vi "Periodic Tasks.vi"(8 "error in":errorcluster) -> ()   [LabVIEW 2016]
doc: "This VI runs in parallel to other tasks. It can contain as many user-defined periodic loops as you need. These can carry out PID or other sorts of timed response."
uses:
  <vilib>/Rock Robotics/WPI/DriverStation/WPI_DriverStationRobotMode2.ctl
  <vilib>/Rock Robotics/WPI/Utilities/WPI_GetSetVariantRefNum.vi
  Robot Global Data.vi
  AutoLeftDrive.vi
  AutoRightDrive.vi
  Target x Location.vi
  AutoModEnable.vi
  AutoProceed.vi
  AutoMod.vi
  <vilib>/Rock Robotics/Network Tables/NT Write Number.vi
  <vilib>/Rock Robotics/WPI/Ultrasonic/WPI_SonarSRF04DigitalRefNum Registry Get.vi
  <vilib>/Rock Robotics/WPI/Ultrasonic/WPI_SonarSRF04DigitalGetRange.vi
panel:
  out "Auto Mod Enable":bool
  out "Target x Location contr":dbl
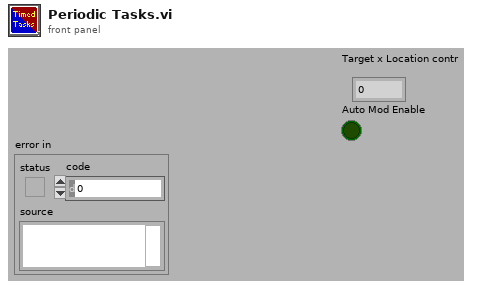
[diagram p1: front panel]
types:
  T1 = typedef "WPI_JoystickDevRef.ctl" = cluster{"Device":T2}
  T2 = typedef "WPI_JoystickDeviceEnum.ctl" = enum16{"USB 0", "USB 1", "USB 2", "USB 3", "USB 4", "USB 5"}
  T3 = typedef "WPI_RobotDriveDevRef.ctl" = cluster{"DevStatus":errorcluster, "Motors[]":T4[], "Square Inputs":bool, "Max Output":dbl}
  T4 = typedef "WPI_MotorControlDeviceRef.ctl" = cluster{"DeviceStatus":errorcluster, "Type":T5, "PWM":cluster{"PWM Channel":T6, "DeadBand":T7}, "CAN":cluster{"Device Number":u8, "SetOutput VI Ref":variant, "GetOutput VI Ref":variant, "Enable VI Ref":variant, "Disable VI Ref":variant, "Data":variant}, "Invert":bool}
  T5 = typedef "WPI_MotorControlType.ctl" = enum16{"PWM", "CAN"}
  T6 = typedef "FPGA_DIOPWMChannel.ctl" = enum8{"PWM 0", "PWM 1", "PWM 2", "PWM 3", "PWM 4", "PWM 5", "PWM 6", "PWM 7", "PWM 8", "PWM 9", "PWM MXP 0", "PWM MXP 1", "PWM MXP 2", "PWM MXP 3", "PWM MXP 4", "PWM MXP 5", "PWM MXP 6", "PWM MXP 7", "PWM MXP 8", "PWM MXP 9", "Invalid"}
  T7 = typedef "WPI_PWMDeadband.ctl" = cluster{"Name":string, "maxPositivePwm":i32, "minPositivePwm":i32, "centerPwm":i32, "maxNegativePwm":i32, "minNegativePwm":i32, "angularRange":u16}
  T8 = typedef "WPI_DriverStationRobotMode2.ctl" = enum16{"Autonomous Disabled", "Autonomous Enabled", "Teleop Disabled", "Teleop Enabled", "Disconnected", "Finish", "Test Disabled", "Test Enabled", "Emergency Stopped"}
  T9 = cluster{"JoystickDevRef":T1, "RobotDriveDevRef":T3}
  T10 = typedef "WPI_GyroDevRef.ctl" = cluster{"DevStatus":errorcluster, "Analog Channel":T11, "Offset":dbl, "Gain (VoltsPerDegree/Second)":dbl, "Gyro Type":enum16{"Analog", "XRS450"}, "Handle":i32, "SPI Bus":T12, "Device Found":bool, "Sample Rate":dbl, "Calibrate On Open":bool}
  T11 = typedef "FPGA_AIChannel.ctl" = enum8{"AI 0", "AI 1", "AI 2", "AI 3", "AI MXP 0", "AI MXP 1", "AI MXP 2", "AI MXP 3", "Invalid"}
  T12 = typedef "spi_bus.ctl" = enum16{"SPI On-Board, CS0", "SPI On-Board, CS1", "SPI On-Board, CS2", "SPI On-Board, CS3", "SPI MXP", "Invalid"}
  T13 = typedef "WPI_UltrasonicDeviceRef.ctl" = cluster{"DevStatus":errorcluster, "Ping Channel":T14, "Echo Channel":T14, "CntIndex":T15}
  T14 = typedef "FPGA_DIOChannel.ctl" = enum8{"DIO 0", "DIO 1", "DIO 2", "DIO 3", "DIO 4", "DIO 5", "DIO 6", "DIO 7", "DIO 8", "DIO 9", "DIO MXP 0", "DIO MXP 1", "DIO MXP 2", "DIO MXP 3", "DIO MXP 4", "DIO MXP 5", "DIO MXP 6", "DIO MXP 7", "DIO MXP 8", "DIO MXP 9", "DIO MXP 10", "DIO MXP 11", "DIO MXP 12", "DIO MXP 13", "DIO MXP 14", "DIO MXP 15", "SPI Port CS1", "SPI Port CS2", "SPI Port CS3", "SPI Port MISO", "SPI Port MOSI", "Invalid"}
  T15 = typedef "FPGA_CounterCtrSystemIndex.ctl" = enum8{"Ctr 0", "Ctr 1", "Ctr 2", "Ctr 3", "Ctr 4", "Ctr 5", "Ctr 6", "Ctr 7", "Invalid"}
  T16 = typedef "WPI_EncoderDevRef.ctl" = cluster{"DevStatus":errorcluster, "EncoderIndex":T17, "CounterIndex":T15, "DistancePerCount":dbl, "Decoding Type":T18}
  T17 = typedef "FPGA_EncoderIdx.ctl" = enum8{"Enc 0", "Enc 1", "Enc 2", "Enc 3", "Enc 4", "Enc 5", "Enc 6", "Enc 7", "Invalid"}
  T18 = typedef "WPI_EncoderType.ctl" = enum16{"1x", "2x", "4x"}
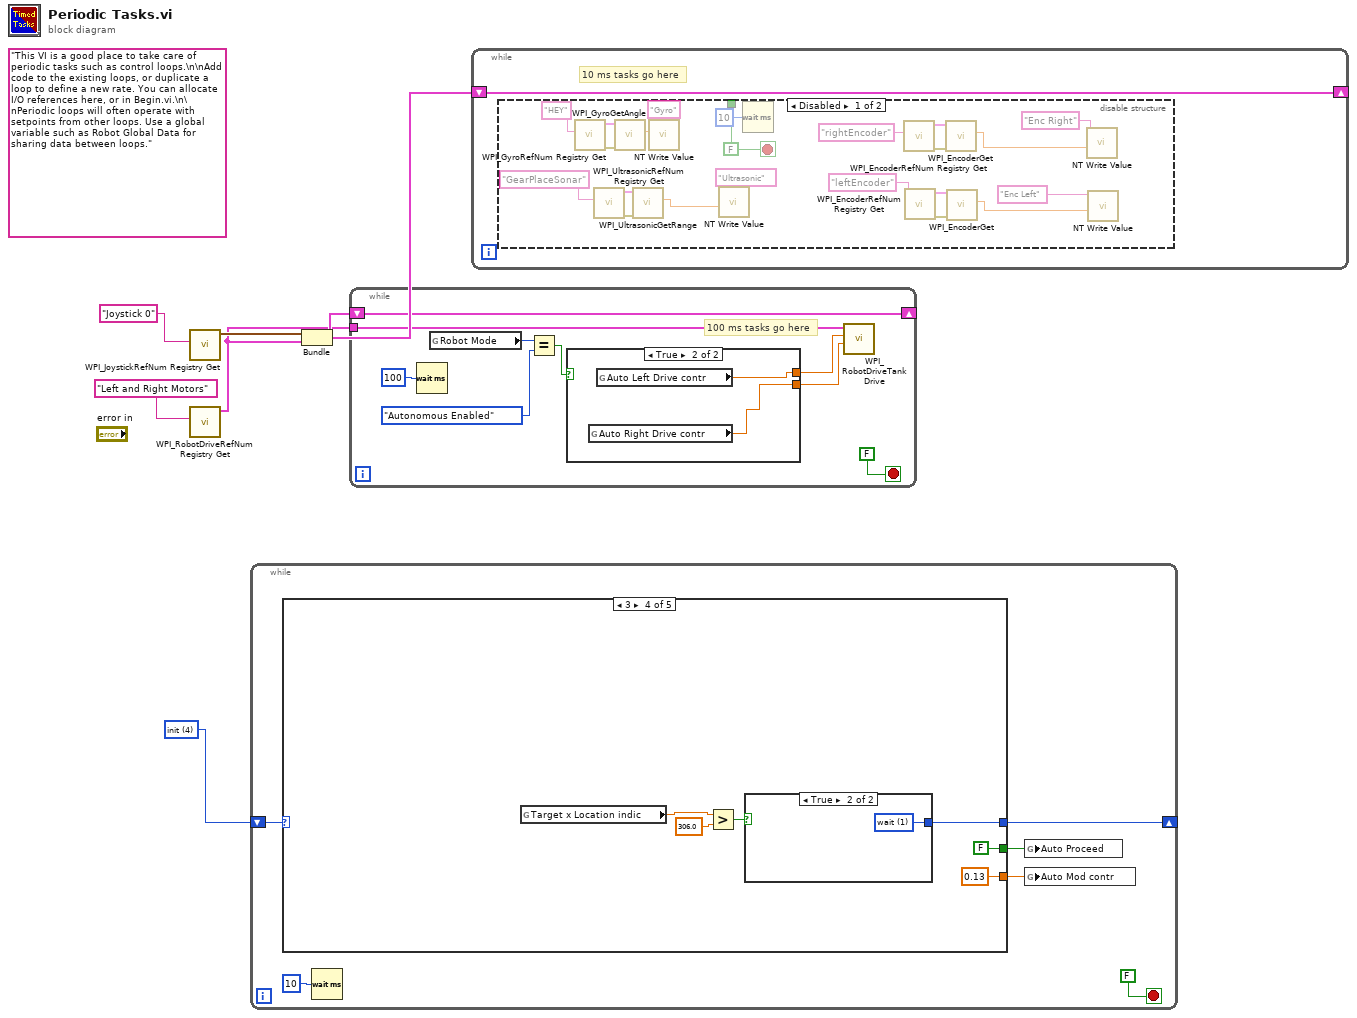
[diagram p0: block diagram]
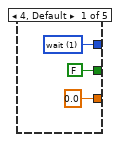
[diagram p2: hidden frame]
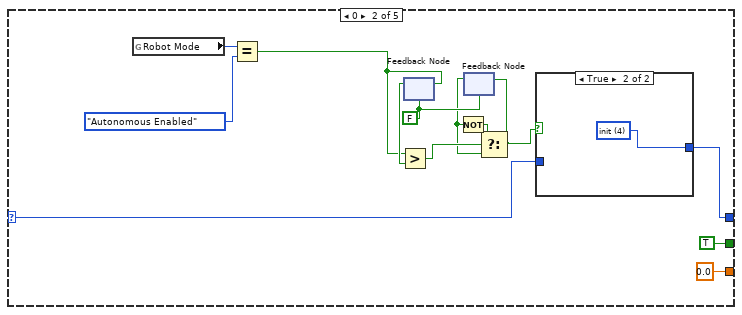
[diagram p3: hidden frame]
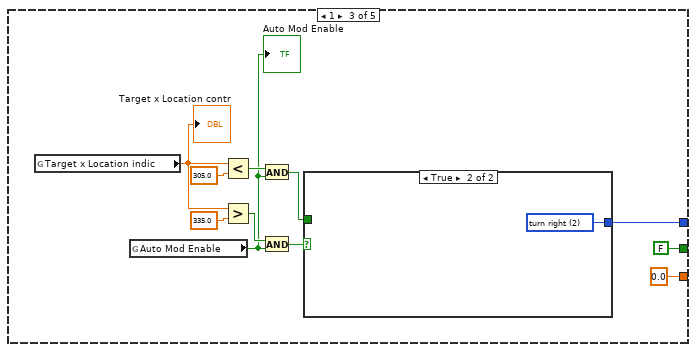
[diagram p5: hidden frame]
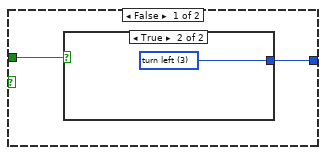
[diagram p6: hidden frame]
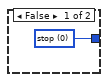
[diagram p7: hidden frame]
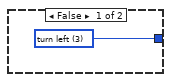
[diagram p8: hidden frame]
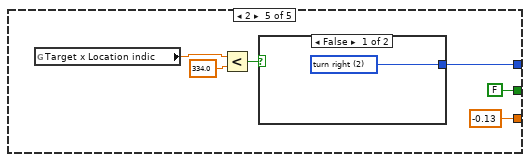
[diagram p9: hidden frame]
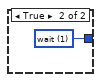
[diagram p10: hidden frame]
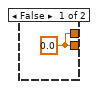
[diagram p11: hidden frame]
diagram:
  w2 = u16 4 items=["stop", "wait", "turn right", "turn left", "init"]
  (unwired) "This VI is a good place to take care of periodic tasks such as control loops.\n\nAdd code to the existing loops, or duplicate a loop to define a new rate. You can allocate I/O references here, or in Begin.vi.\n\nPeriodic loops will often operate with setpoints from other loops. Use a global variable such as Robot Global Data for sharing data between loops."
  n1 = call <vilib>:"WPI_JoystickRefNum Registry Get.vi"("refnum name"="Joystick 0") -> ("JoystickDevRef"=w4:T1)  [unwired: 1 in, 9 out]
  n2 = call <vilib>:"WPI_RobotDriveRefNum Registry Get.vi"("refnum name"="Left and Right Motors") -> ("RobotDriveDevRef"=w1:T3)  [unwired: 1 in, 9 out]
  n3 = while {
    shift-right: [w8] -> _
    shift-left: w2 -> [w7]
    stop <- FALSE stop-if-true
    n4 = case shown="3" w7 {
      selector: w7 -> [_ w16 _ _ _]
      tunnel: [0.0 0.0 0.0 0.13 -0.13] -> w10
      tunnel: [FALSE TRUE FALSE FALSE FALSE] -> w9
      tunnel: [w13 w17 w33 w49 w57] -> w8
      frame 4, Default {
        w13 = u16 1 items=["stop", "wait", "turn right", "turn left", "init"]
      }
      frame 0 {
        w22 = FALSE ("Boolean")
        n5 = global read "Robot Global Data.vi" "Robot Mode"() -> (w25:T8)
        n6 = Equal?(x=w25, y=WPI_DriverStationRobotMode2."Autonomous Enabled" ("Robot Mode")) -> (x = y?=w19:bool)
        n7 = feedback #1(w22) -> (w24:bool)
        n8 = Greater?(x=w19, y=w24) -> (0:w23:bool)
        n9 = feedback-in #1(w19) -> ()
        n10 = feedback #2(w22) -> (w21:bool)
        n11 = Not(x=w21) -> (.not. x?=w20:bool)
        n12 = Select(t=w20, s=w23, f=w21) -> (s? t:f=w18:bool)
        n13 = feedback-in #2(w18) -> ()
        n14 = case shown="True" w18 {
          tunnel: [w29 w30] -> w17
          tunnel: w16 -> [w29 _]
          frame False {
          }
          frame True {
            w30 = u16 4 items=["stop", "wait", "turn right", "turn left", "init"]
          }
        }
      }
      frame 1 {
        n15 = global read "Target x Location.vi" "Target x Location indic"() -> (w40:dbl)
        "Target x Location contr" <- w40
        n16 = global read "AutoModEnable.vi" "Auto Mod Enable"() -> (w36:bool)
        "Auto Mod Enable" <- w36
        n17 = Less?(x=w40, y=305.0) -> (x < y?=w37:bool)
        n18 = Greater?(x=w40, y=335.0) -> (0:w38:bool)
        n19 = And(x=w37, y=w36) -> (x .and. y?=w34:bool)
        n20 = And(x=w38, y=w36) -> (x .and. y?=w35:bool)
        n21 = case shown="True" w35 {
          tunnel: w34 -> [w43 _]
          tunnel: [w42 w46] -> w33
          frame False {
            n22 = case shown="True" w43 {
              tunnel: [w44 w45] -> w42
              frame False {
                w44 = u16 0 items=["stop", "wait", "turn right", "turn left", "init"]
              }
              frame True {
                w45 = u16 3 items=["stop", "wait", "turn right", "turn left", "init"]
              }
            }
          }
          frame True {
            w46 = u16 2 items=["stop", "wait", "turn right", "turn left", "init"]
          }
        }
      }
      frame 3 {
        n23 = global read "Target x Location.vi" "Target x Location indic"() -> (w52:dbl)
        n24 = Greater?(x=w52, y=306.0) -> (0:w50:bool)
        n25 = case shown="True" w50 {
          tunnel: [w53 w54] -> w49
          frame False {
            w53 = u16 3 items=["stop", "wait", "turn right", "turn left", "init"]
          }
          frame True {
            w54 = u16 1 items=["stop", "wait", "turn right", "turn left", "init"]
          }
        }
      }
      frame 2 {
        n26 = global read "Target x Location.vi" "Target x Location indic"() -> (w60:dbl)
        n27 = Less?(x=w60, y=334.0) -> (x < y?=w58:bool)
        n28 = case shown="False" w58 {
          tunnel: [w61 w62] -> w57
          frame False {
            w61 = u16 2 items=["stop", "wait", "turn right", "turn left", "init"]
          }
          frame True {
            w62 = u16 1 items=["stop", "wait", "turn right", "turn left", "init"]
          }
        }
      }
    }
    n29 = Wait (ms)(milliseconds to wait=u32 10) -> ()  [unwired: 1 out]
    n30 = global write "AutoProceed.vi" "Auto Proceed"(w9) -> ()
    n31 = global write "AutoMod.vi" "Auto Mod contr"(w10) -> ()
  }
  n32 = Bundle("JoystickDevRef"=w4, "RobotDriveDevRef"=w1) -> (w3:T9)  [unwired: 1 out]
  n33 = while {
    shift-right: [w69] -> _
    shift-left: w3 -> [w69]
    tunnel: w1 -> [w63]
    stop <- FALSE stop-if-true
    # "100 ms tasks go here"
    n34 = Wait (ms)(milliseconds to wait=u32 100) -> ()  [unwired: 1 out]
    n35 = global read "Robot Global Data.vi" "Robot Mode"() -> (w66:T8)
    n36 = Equal?(x=w66, y=WPI_DriverStationRobotMode2."Autonomous Enabled" ("Robot Mode")) -> (x = y?=w68:bool)
    n37 = case shown="True" w68 {
      tunnel: [w72 w73] -> w65
      tunnel: [w72 w74] -> w64
      frame False {
        w72 = 0.0
      }
      frame True {
        n38 = global read "AutoRightDrive.vi" "Auto Right Drive contr"() -> (w74:dbl)
        n39 = global read "AutoLeftDrive.vi" "Auto Left Drive contr"() -> (w73:dbl)
      }
    }
    n40 = call <vilib>:"WPI_RobotDriveTankDrive.vi"("Right axis value"=w64, "Left axis value"=w65, "RobotDriveDevRef"=w63) -> ()  [unwired: 6 in, 3 out]
  }
  n41 = while {
    shift-right: [w75] -> _
    shift-left: w3 -> [w75]
    stop <- w76 stop-if-true
    # "10 ms tasks go here"
    n42 = disable-structure shown="Disabled" {
      disable-tunnel: [FALSE _] -> w76
      frame Disabled {
        n43 = call <vilib>:"WPI_GyroRefNum Registry Get.vi"("refnum name"="HEY") -> ("error out"=w88:errorcluster, "GyroDevRef"=w89:T10)  [unwired: 9 in]
        n44 = call-poly <vilib>:"WPI_UltrasonicRefNum Registry Get.vi"("refnum name"="GearPlaceSonar") -> ("error out"=w92:errorcluster, "SonarSRF04DevRef"=w93:T13)  [unwired: 9 in]
        n45 = call <vilib>:"WPI_GyroGetAngle.vi"("error in"=w88, "GyroDevRef"=w89) -> ("Angle"=w91:dbl)  [unwired: 5 in, 4 out]
        n46 = call-poly <vilib>:"WPI_UltrasonicGetRange.vi"("error in (no error)"=w92, "SonarSRF04DevRef"=w93) -> ("Distance"=w94:dbl)  [unwired: 7 in, 2 out]
        n47 = call-poly <vilib>:"NT Write Value.vi"("Numeric"=w91, "Name"="Gyro") -> ()  [unwired: 9 in, 1 out]
        n48 = call-poly <vilib>:"NT Write Value.vi"("Numeric"=w94, "Name"="Ultrasonic") -> ()  [unwired: 9 in, 1 out]
        n49 = Wait (ms)(milliseconds to wait=u32 10) -> ()  [unwired: 1 out]
        n50 = call <vilib>:"WPI_EncoderRefNum Registry Get.vi"("refnum name"="rightEncoder") -> ("error out"=w82:errorcluster, "EncoderDevRef"=w81:T16)  [unwired: 9 in]
        n51 = call <vilib>:"WPI_EncoderRefNum Registry Get.vi"("refnum name"="leftEncoder") -> ("error out"=w80:errorcluster, "EncoderDevRef"=w79:T16)  [unwired: 9 in]
        n52 = call <vilib>:"WPI_EncoderGet.vi"("error in (no error)"=w82, "EncoderDevRef"=w81) -> ("Distance"=w78:dbl)  [unwired: 4 in, 5 out]
        n53 = call <vilib>:"WPI_EncoderGet.vi"("error in (no error)"=w80, "EncoderDevRef"=w79) -> ("Distance"=w77:dbl)  [unwired: 4 in, 5 out]
        n54 = call-poly <vilib>:"NT Write Value.vi"("Numeric"=w78, "Name"="Enc Right") -> ()  [unwired: 9 in, 1 out]
        n55 = call-poly <vilib>:"NT Write Value.vi"("Numeric"=w77, "Name"="Enc Left") -> ()  [unwired: 9 in, 1 out]
      }
      frame Enabled {
      }
    }
  }
